vi "patch_add.vi"(8 "signal in":waveform(dbl), 9 "phase":dbl format="%.2p", 10 "amplitude":dbl=1.0 format="%0.2p", 11 "image time":dbl=10.0 format="%0.2p") -> (0 "signal out":waveform(dbl), 4 "patch freq":dbl)   [LabVIEW 2021]
uses:
  <vilib>/Waveform/WDTOps.llb/WDT Number of Waveform Samples DBL.vi
  <vilib>/measure/NI_MABase.lvlib
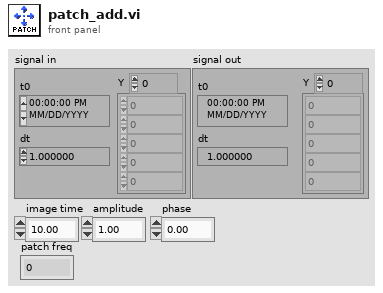
[diagram p1: front panel]
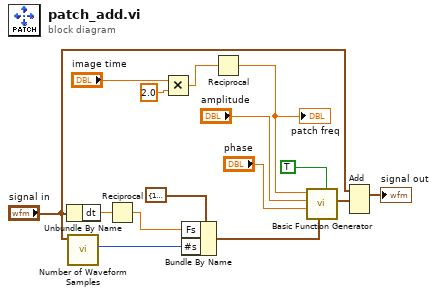
[diagram p0: block diagram]
diagram:
  n1 = Unbundle By Name("signal in") -> ("dt"=w10:dbl)
  n2 = call-poly <vilib>:"Number of Waveform Samples.vi"("waveform in"="signal in") -> ("number of samples"=w7:i32)  [unwired: 8 in, 2 out]
  n3 = Reciprocal(x=w10) -> (1/x=w9:dbl)
  n4 = Multiply(x="image time", y=2.0) -> (x*y=w2:dbl)
  n5 = Bundle By Name(cluster=cluster{"Fs":dbl, "#s":dbl} {"Fs"=1000.0, "#s"=1000.0} ("sampling info"), "Fs"=w9, "#s"=w7) -> (w6:cluster{"Fs":dbl, "#s":dbl})
  n6 = Reciprocal(x=w2) -> (1/x=w1:dbl)
  "patch freq" <- w1
  n7 = call <vilib>:"Basic Function Generator.vi"("reset signal"=TRUE, "sampling info"=w6, "phase"="phase", "amplitude"="amplitude", "frequency"=w1) -> ("signal out"=w15:waveform(dbl))  [unwired: 4 in, 2 out]
  n8 = Add(1:w15, 2:"signal in") -> (0:→"signal out":waveform(dbl))  [unwired: 1 in, 1 out]
